vi "Destructor.vi"(8 "error in":errorcluster, 11 "Baseline Mocon \npiD-Tech plus in":refnum<class "Baseline Mocon piD-Tech plus.lvclass">) -> (0 "error out":errorcluster, 3 "Baseline Mocon \npiD-Tech plus out":refnum<class "Baseline Mocon piD-Tech plus.lvclass">)   [LabVIEW 2011, in "Baseline Mocon piD-Tech plus.lvclass"]
uses:
  Baseline Mocon piD-Tech plus.lvclass
  Baseline Mocon piD-Tech plus.lvclass/Baseline Mocon piD-Tech plus.ctl
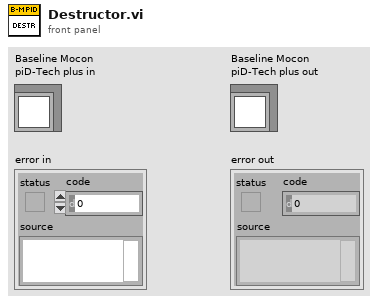
[diagram p1: front panel]
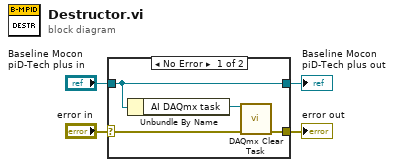
[diagram p0: block diagram]
diagram:
  n1 = case shown="No Error" "error in" {
    selector: "error in" -> [w7 w10]
    tunnel: [w6 w10] -> w3
    tunnel: [w5 w9] -> w1
    tunnel: "Baseline Mocon \npiD-Tech plus in" -> [w5 w9]
    frame No Error {
      n2 = Unbundle By Name(w5) -> ("AI DAQmx task"=w8:refnum<k21>)
      n3 = call <vilib>:"DAQmx Clear Task.vi"("task in"=w8, "error in"=w7) -> ("error out"=w6:errorcluster)  [unwired: 13 in]
    }
    frame Error {
    }
  }
  "error out" <- w3
  "Baseline Mocon \npiD-Tech plus out" <- w1
